vi "Sensor Calibration.vi"(7 "I2C Channel":u8, 8 "error in (no error)":errorcluster, 10 "Calibration Time (s)":u32, 11 "LINX Resource In":T1) -> (0 "error out":errorcluster, 3 "LINX Resource Out":T1)   [LabVIEW 2014, in "LMH-LINX.lvlib" / "HMC6352.lvlib"]
uses:
  <vilib>/MakerHub/LINX/Public/Sensors/Orientation/Compass/HMC6352/HMC6352.lvlib
  <vilib>/MakerHub/LINX/Private/Type Defs/LINX Ref.ctl
  <vilib>/MakerHub/LINX/Private/Type Defs/Platform.ctl
  <vilib>/MakerHub/LINX/Private/Type Defs/Interface.ctl
  <vilib>/MakerHub/LINX/Private/Device/Type Defs/LINX Device Config.ctl
  <vilib>/MakerHub/LINX/Private/Device/Type Defs/TCP Config.ctl
  <vilib>/MakerHub/LINX/Private/Device/Type Defs/Channels.ctl
  <vilib>/MakerHub/LINX/Private/Local IO/LinxI2cWrite.vi
  <vilib>/MakerHub/LINX/Public/Utilities/Check Channel.vi
  <vilib>/MakerHub/LINX/Private/Utilties/Generate Error.vi
  <vilib>/MakerHub/LINX/LMH-LINX.lvlib
  <vilib>/MakerHub/LINX/Private/Device/Device.lvlib
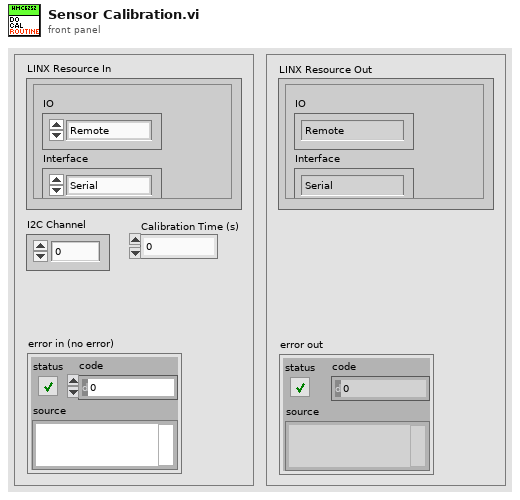
[diagram p1: front panel]
types:
  T1 = typedef "LMH-LINX.lvlib/LINX Ref.ctl" = cluster{"IO":T2, "Interface":T3, "LINX Device Config":T4}
  T2 = typedef "LMH-LINX.lvlib/Platform.ctl" = enum16{"Remote", "Local"}
  T3 = typedef "LMH-LINX.lvlib/Interface.ctl" = enum16{"Serial", "TCP"}
  T4 = typedef "LMH-LINX.lvlib/Device.lvlib/LINX Device Config.ctl" = cluster{"Interface":T3, "COM Port":refnum<visa-resource-name>, "TCP Configuration":T5, "Device Family":u8, "Device ID":u8, "Device Name":string, "TCP Ref":refnum<k5>, "Channels":T6}
  T5 = typedef "LMH-LINX.lvlib/Device.lvlib/TCP Config.ctl" = cluster{"IP Address":string, "Port":u16}
  T6 = typedef "LMH-LINX.lvlib/Channels.ctl" = cluster{"DI":u8[], "DO":u8[], "AI":u8[], "AO":u8[], "PWM":u8[], "QE":u8[], "UART":u8[], "I2C 2":u8[], "SPI":u8[], "CAN":u8[], "Servo":u8[], "AI Ref (V)":dbl, "AI Resolution (Bits)":u8, "AO Ref (V)":dbl, "AO Resolution (Bits)":u8}
  T7 = enum8{"Enter Calibration", "Wait", "Exit Calibration"}
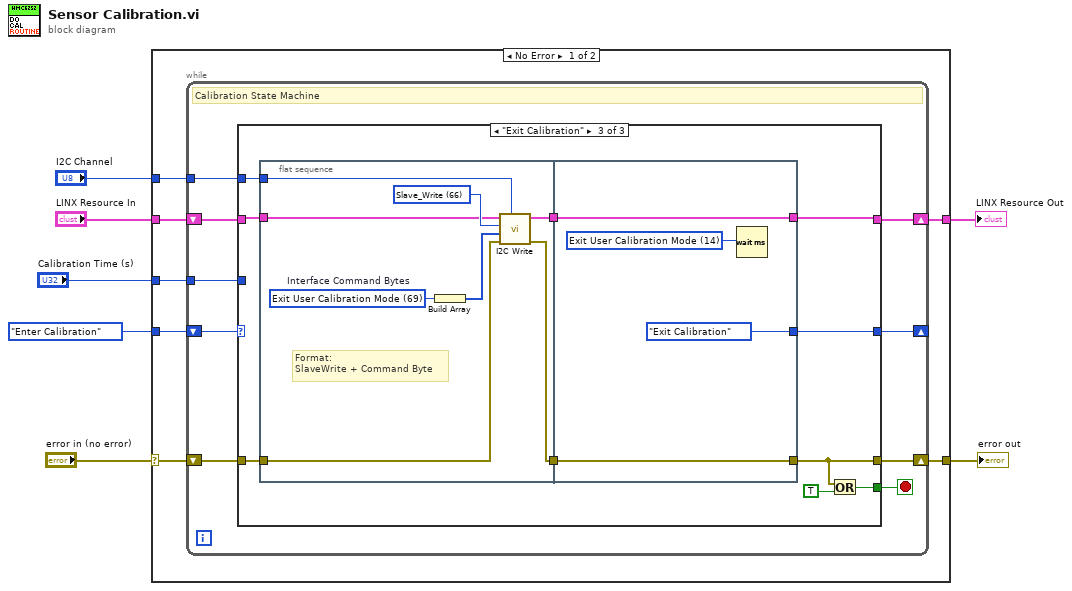
[diagram p0: block diagram]
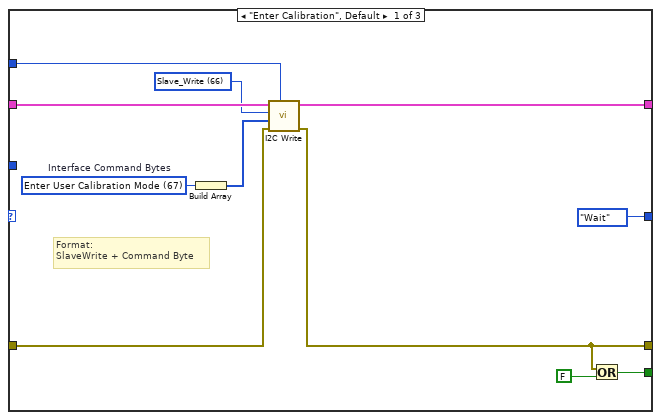
[diagram p2: hidden frame]
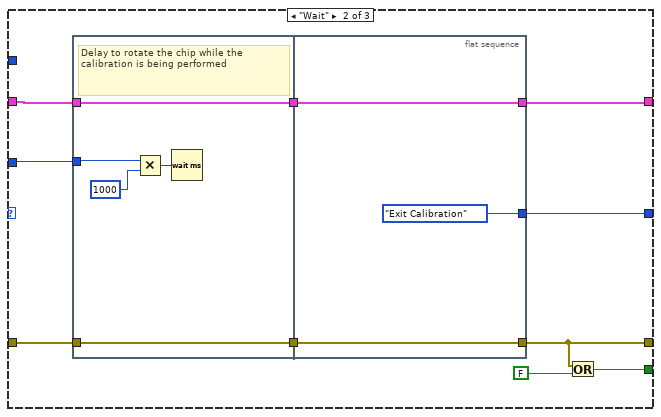
[diagram p3: hidden frame]
diagram:
  n1 = case shown="No Error" "error in (no error)" {
    selector: "error in (no error)" -> [w12 w76]
    tunnel: [w10 w76] -> w6
    tunnel: "LINX Resource In" -> [w14 w75]
    tunnel: "I2C Channel" -> [w13 _]
    tunnel: [w11 w75] -> w3
    tunnel: T7."Enter Calibration" ("Calibration State") -> [w9 _]
    tunnel: "Calibration Time (s)" -> [w8 _]
    frame No Error {
      n2 = while {
        tunnel: w13 -> [w22]
        shift-right: [w20] -> w11
        shift-left: w14 -> [w23]
        shift-right: [w19] -> w10
        shift-left: w12 -> [w21]
        shift-right: [w16] -> _
        shift-left: w9 -> [w18]
        tunnel: w8 -> [w15]
        stop <- w17 stop-if-true
        # "Calibration State Machine"
        n3 = case shown="\"Exit Calibration\"" w18 {
          tunnel: w23 -> [w34 w39 w61]
          tunnel: w22 -> [w33 _ w62]
          tunnel: w21 -> [w32 w42 w60]
          tunnel: [w31 w38 w55] -> w20
          tunnel: [w24 w35 w53] -> w19
          tunnel: [w26 w37 w59] -> w17
          tunnel: [T7."Wait" ("Calibration State") w43 w57] -> w16
          tunnel: w15 -> [_ w44 _]
          frame "Enter Calibration", Default {
            w29 = u8 67 items=["Write to EEPROM"=119, "Read from EEPROM"=114, "Write to RAM Register"=71, "Read from RAM Register"=103, "Enter Sleep Mode"=83, "Exit Sleep Mode"=87, "Update Bridge Offsets (Set/Reset)"=79, "Enter User Calibration Mode"=67, "Exit User Calibration Mode"=69, "Save Operation Mode to EEPROM"=76, "J_Who_am_i"=117, "Get Data/Calculate New Heading"=65]  # Interface Command Bytes
            w28 = u8 66 items=["Slave_Write"=66, "Slave_Read"=67] ("HMC6352 Slave Address")
            # "Format:\nSlaveWrite + Command Byte"
            n4 = Build Array(w29) -> (w30:u8[])
            n5 = call <vilib>:"I2C Write.vi"("I2C Channel"=w33, "Error In"=w32, "Data"=w30, "I2C Slave Address (0)"=w28, "LINX Resource"=w34) -> ("Error Out"=w24:errorcluster, "LINX Resource"=w31:T1)  [unwired: 5 in]
            n6 = Or(x=w24, y=FALSE) -> (x .or. y?=w26:bool)
          }
          frame "Wait" {
            n7 = flat-sequence {
              tunnel: w44 -> [w47]
              tunnel: w42 -> [w49]
              tunnel: [w49] -> w41
              tunnel: [w48] -> w40
              tunnel: w39 -> [w48]
              tunnel: [T7."Exit Calibration" ("Calibration State")] -> w43
              tunnel: w41 -> [w51]
              tunnel: [w51] -> w35
              tunnel: w40 -> [w50]
              tunnel: [w50] -> w38
              frame #0 {
                # "Delay to rotate the chip while the calibration is being performed"
                n8 = Multiply(x=w47, y=u32 1000) -> (x*y=w46:u32)
                n9 = Wait (ms)(milliseconds to wait=w46) -> ()  [unwired: 1 out]
              }
              frame #1 {
              }
            }
            n10 = Or(x=w35, y=FALSE) -> (x .or. y?=w37:bool)
          }
          frame "Exit Calibration" {
            n11 = flat-sequence {
              tunnel: w62 -> [w67]
              tunnel: w61 -> [w66]
              tunnel: w60 -> [w65]
              tunnel: [w64] -> w58
              tunnel: [w63] -> w56
              tunnel: [w74] -> w53
              tunnel: w58 -> [w74]
              tunnel: [T7."Exit Calibration" ("Calibration State")] -> w57
              tunnel: [w72] -> w55
              tunnel: w56 -> [w72]
              frame #0 {
                w69 = u8 69 items=["Write to EEPROM"=119, "Read from EEPROM"=114, "Write to RAM Register"=71, "Read from RAM Register"=103, "Enter Sleep Mode"=83, "Exit Sleep Mode"=87, "Update Bridge Offsets (Set/Reset)"=79, "Enter User Calibration Mode"=67, "Exit User Calibration Mode"=69, "Save Operation Mode to EEPROM"=76, "J_Who_am_i"=117, "Get Data/Calculate New Heading"=65]  # Interface Command Bytes
                w68 = u8 66 items=["Slave_Write"=66, "Slave_Read"=67] ("HMC6352 Slave Address")
                # "Format:\nSlaveWrite + Command Byte"
                n12 = Build Array(w69) -> (w70:u8[])
                n13 = call <vilib>:"I2C Write.vi"("I2C Channel"=w67, "Error In"=w65, "Data"=w70, "I2C Slave Address (0)"=w68, "LINX Resource"=w66) -> ("Error Out"=w64:errorcluster, "LINX Resource"=w63:T1)  [unwired: 5 in]
              }
              frame #1 {
                w71 = u32 14 items=["Update Bridge Offsets"=6, "Exit User Calibration Mode"=14, "Get New Heading"=7] ("Command Time Delays (ms)")
                n14 = Wait (ms)(milliseconds to wait=w71) -> ()  [unwired: 1 out]
              }
            }
            n15 = Or(x=w53, y=TRUE) -> (x .or. y?=w59:bool)
          }
        }
      }
    }
    frame Error {
    }
  }
  "error out" <- w6
  "LINX Resource Out" <- w3
